vi "Drive Encoder.vi"(10 "Distance Back":dbl=55.0 format="%.2f", 11 "Execute?":bool=TRUE) -> (3 "Done":bool=TRUE)   [LabVIEW 2012]
uses:
  <vilib>/addons/control/pid/pid.llb/PID (DBL).vi
  <vilib>/addons/control/pid/NI_PID_pid.lvlib
panel:
  in  "Left gains":T1={"proportional gain (Kc)"=0.015, "integral time (Ti, min)"=0.0, "derivative time (Td, min)"=0.0}
  out "Right":bool=TRUE
  out "Left":bool=TRUE
  out "Right":dbl=0.2956416378701198
  out "Left":dbl=-0.2957320237980065
  in  "Right gains":T1={"proportional gain (Kc)"=0.05, "integral time (Ti, min)"=0.0, "derivative time (Td, min)"=0.0}
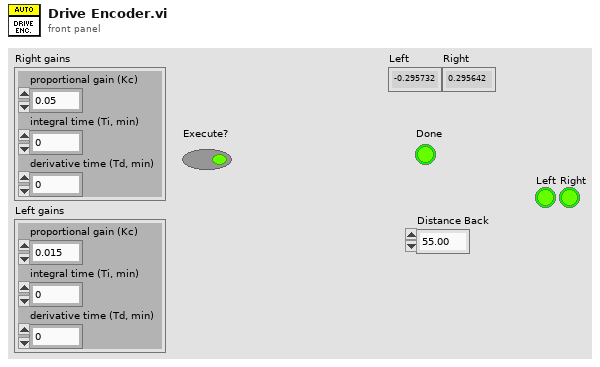
[diagram p1: front panel]
types:
  T1 = cluster{"proportional gain (Kc)":dbl, "integral time (Ti, min)":dbl, "derivative time (Td, min)":dbl}
  T2 = typedef "WPI_MotorControlDeviceRef.ctl" = cluster{"DeviceStatus":errorcluster, "Type":enum16{"PWM", "CAN"}, "PWM":cluster{"Digital Module":T3, "PWM Channel":T4, "DeadBand":T5}, "CAN":cluster{"Device Number":u8, "Control Mode":T6, "Semaphore":T7, "Max Vout":dbl}, "Invert":bool, "TransformRef":T8, "InvTransformRef":T8}
  T3 = typedef "FPGA_TypedefDigitalModule.ctl" = enum16{"Digital Module 1", "Digital Module 2"}
  T4 = typedef "FPGA_DIOPWMChannel.ctl" = enum8{"PWM 1", "PWM 2", "PWM 3", "PWM 4", "PWM 5", "PWM 6", "PWM 7", "PWM 8", "PWM 9", "PWM 10", "Invalid"}
  T5 = typedef "WPI_PWMDeadband.ctl" = cluster{"Name":string, "maxPositivePwm":i32, "minPositivePwm":i32, "centerPwm":i32, "maxNegativePwm":i32, "minNegativePwm":i32, "angularRange":u16}
  T6 = typedef "WPI_CANJaguar_ControlMode.ctl" = enum8{"Percent VBus", "Current", "Speed", "Position", "Voltage"}
  T7 = typedef "Semaphore RefNum" = refnum<k1>
  T8 = typedef "WPI_PWMTransform_ConPane.ctl" = refnum<vi>
  T9 = typedef "WPI_EncoderDevRef.ctl" = cluster{"DevStatus":errorcluster, "EncoderIndex":T10, "CounterIndex":T11, "DistancePerCount":dbl, "Decoding Type":T12}
  T10 = typedef "FPGA_EncoderIdx.ctl" = enum8{"Enc 0", "Enc 1", "Enc 2", "Enc 3", "Invalid"}
  T11 = typedef "FPGA_CounterCtrSystemIndex.ctl" = enum8{"Ctr 0", "Ctr 1", "Ctr 2", "Ctr 3", "Ctr 4", "Ctr 5", "Ctr 6", "Ctr 7", "Invalid"}
  T12 = typedef "WPI_EncoderType.ctl" = enum16{"1x", "2x", "4x"}
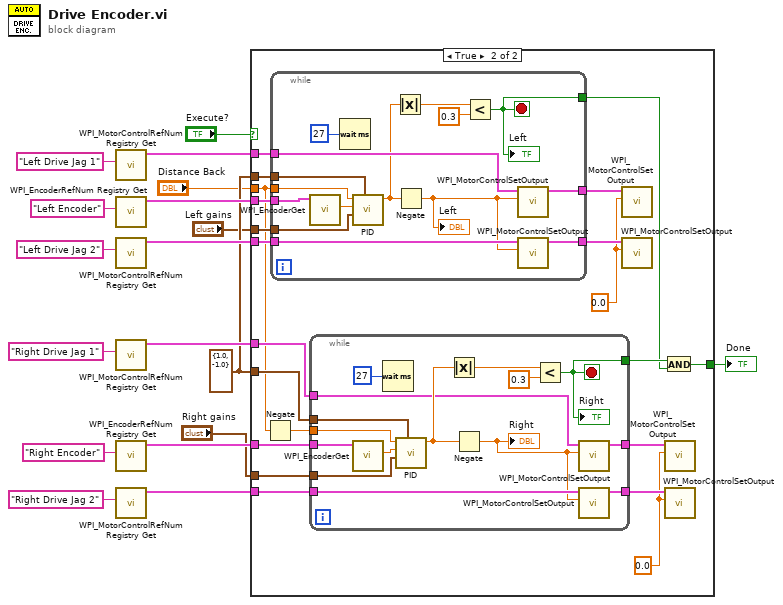
[diagram p0: block diagram]
diagram:
  w4 = cluster{"output high":dbl, "output low":dbl} {"output high"=1.0, "output low"=-1.0} ("output range")
  n1 = call <vilib>:"WPI_MotorControlRefNum Registry Get.vi"("refnum name"="Left Drive Jag 1") -> ("MotorControlDevRef"=w6:T2)  [unwired: 9 in, 1 out]
  n2 = call <vilib>:"WPI_EncoderRefNum Registry Get.vi"("refnum name"="Left Encoder") -> ("EncoderDevRef"=w14:T9)  [unwired: 9 in, 1 out]
  n3 = call <vilib>:"WPI_MotorControlRefNum Registry Get.vi"("refnum name"="Left Drive Jag 2") -> ("MotorControlDevRef"=w5:T2)  [unwired: 9 in, 1 out]
  n4 = call <vilib>:"WPI_MotorControlRefNum Registry Get.vi"("refnum name"="Right Drive Jag 1") -> ("MotorControlDevRef"=w8:T2)  [unwired: 9 in, 1 out]
  n5 = call <vilib>:"WPI_EncoderRefNum Registry Get.vi"("refnum name"="Right Encoder") -> ("EncoderDevRef"=w13:T9)  [unwired: 9 in, 1 out]
  n6 = call <vilib>:"WPI_MotorControlRefNum Registry Get.vi"("refnum name"="Right Drive Jag 2") -> ("MotorControlDevRef"=w7:T2)  [unwired: 9 in, 1 out]
  n7 = case shown="True" "Execute?" {
    selector: "Execute?" -> [w19 _]
    tunnel: [w19 w32] -> w15
    tunnel: w14 -> [_ w40]
    tunnel: w13 -> [_ w39]
    tunnel: "Distance Back" -> [_ w27]
    tunnel: w8 -> [_ w38]
    tunnel: w7 -> [_ w37]
    tunnel: w6 -> [_ w36]
    tunnel: w5 -> [_ w35]
    tunnel: "Right gains" -> [_ w31]
    tunnel: "Left gains" -> [_ w30]
    tunnel: w4 -> [_ w29]
    tunnel: w4 -> [_ w28]
    frame False {
    }
    frame True {
      w20 = 0.0 ("Output")
      w21 = 0.0 ("Output")
      n8 = Negate(x=w27) -> (-x=w26:dbl)
      n9 = while {
        tunnel: w40 -> [w70]
        tunnel: w27 -> [w68]
        tunnel: w36 -> [w64]
        tunnel: w35 -> [w63]
        tunnel: [w61] -> w33
        tunnel: w30 -> [w60]
        tunnel: w28 -> [w59]
        tunnel: [w57] -> w25
        tunnel: [w56] -> w24
        stop <- w61 stop-if-true
        n10 = call <vilib>:"WPI_EncoderGet.vi"("EncoderDevRef"=w70) -> ("Distance"=w69:dbl)  [unwired: 5 in, 5 out]
        n11 = Wait (ms)(milliseconds to wait=u32 27) -> ()  [unwired: 1 out]
        n12 = call-poly <vilib>:"PID.vi"("output range"=w59, "PID gains"=w60, "process variable"=w69, "setpoint"=w68) -> ("output"=w62:dbl)  [unwired: 6 in, 1 out]
        n13 = Absolute Value(x=w62) -> (abs(x)=w66:dbl)
        n14 = Negate(x=w62) -> (-x=w58:dbl)
        "Left" <- w58
        n15 = Less?(x=w66, y=0.3) -> (x < y?=w61:bool)
        "Left" <- w61
        n16 = call <vilib>:"WPI_MotorControlSetOutput.vi"("Output"=w58, "MotorControlDevRef"=w64) -> ("MotorControlDevRef"=w57:T2)  [unwired: 7 in, 2 out]
        n17 = call <vilib>:"WPI_MotorControlSetOutput.vi"("Output"=w58, "MotorControlDevRef"=w63) -> ("MotorControlDevRef"=w56:T2)  [unwired: 7 in, 2 out]
      }
      n18 = while {
        tunnel: w39 -> [w55]
        tunnel: w26 -> [w52]
        tunnel: w38 -> [w48]
        tunnel: w37 -> [w47]
        tunnel: [w46] -> w34
        tunnel: w31 -> [w45]
        tunnel: w29 -> [w44]
        tunnel: [w42] -> w23
        tunnel: [w41] -> w22
        stop <- w46 stop-if-true
        n19 = call <vilib>:"WPI_EncoderGet.vi"("EncoderDevRef"=w55) -> ("Distance"=w54:dbl)  [unwired: 5 in, 5 out]
        n20 = Wait (ms)(milliseconds to wait=u32 27) -> ()  [unwired: 1 out]
        n21 = call-poly <vilib>:"PID.vi"("output range"=w44, "PID gains"=w45, "process variable"=w54, "setpoint"=w52) -> ("output"=w49:dbl)  [unwired: 6 in, 1 out]
        n22 = Absolute Value(x=w49) -> (abs(x)=w50:dbl)
        n23 = Negate(x=w49) -> (-x=w43:dbl)
        "Right" <- w43
        n24 = Less?(x=w50, y=0.3) -> (x < y?=w46:bool)
        "Right" <- w46
        n25 = call <vilib>:"WPI_MotorControlSetOutput.vi"("Output"=w43, "MotorControlDevRef"=w48) -> ("MotorControlDevRef"=w42:T2)  [unwired: 7 in, 2 out]
        n26 = call <vilib>:"WPI_MotorControlSetOutput.vi"("Output"=w43, "MotorControlDevRef"=w47) -> ("MotorControlDevRef"=w41:T2)  [unwired: 7 in, 2 out]
      }
      n27 = call <vilib>:"WPI_MotorControlSetOutput.vi"("Output"=w20, "MotorControlDevRef"=w25) -> ()  [unwired: 7 in, 3 out]
      n28 = call <vilib>:"WPI_MotorControlSetOutput.vi"("Output"=w20, "MotorControlDevRef"=w24) -> ()  [unwired: 7 in, 3 out]
      n29 = And(x=w34, y=w33) -> (x .and. y?=w32:bool)
      n30 = call <vilib>:"WPI_MotorControlSetOutput.vi"("Output"=w21, "MotorControlDevRef"=w23) -> ()  [unwired: 7 in, 3 out]
      n31 = call <vilib>:"WPI_MotorControlSetOutput.vi"("Output"=w21, "MotorControlDevRef"=w22) -> ()  [unwired: 7 in, 3 out]
    }
  }
  "Done" <- w15
